vi "Prefilter_60Hz_Notch.vi"(8 "error in (no error)":errorcluster, 10 "Array in":waveform(dbl)[](array[waveform])) -> (0 "error out":errorcluster, 2 "Array out":waveform(dbl)[](array[waveform]))   [LabVIEW 2016, in "LockinDAQ.lvclass"]
uses:
  LockinDAQ.lvclass
  <vilib>/addons/Digital Filter Design/Design.llb/DFD IIR Notch Peak Design by Q.vi
  <vilib>/addons/Digital Filter Design/Process.llb/DFD Filtering (Wfm NChan).vi
  <vilib>/addons/Digital Filter Design/NI_DigFilterLicensed.lvlib
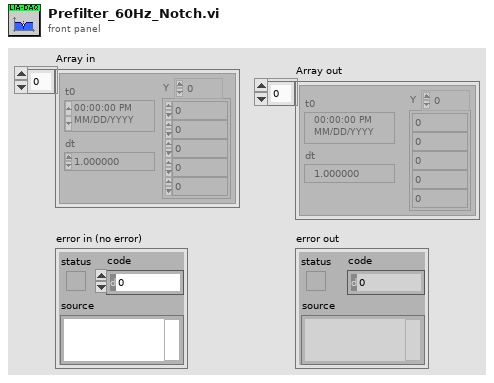
[diagram p1: front panel]
types:
  T1 = typedef "NI_DigFilterLicensed.lvlib/DFD Filter Obj.ctl" = cluster{"mSRate_Fs":dbl, "mSRate_Version":string, "mSRate_Comments":string, "mSRate_OrgCoef":T2, "mSRate_CurCoef":T2, "mSRate_Quantized?":bool, "mSRate_QCoef":T2, "mSRate_QSettings":T4[], "mSRate_Order":i32, "mSRate_Scaling":cluster{"mSRate_ScaleByPowerOf2?":bool, "mSRate_ScaleType":T6}}
  T2 = typedef "NI_DigFilterLicensed.lvlib/DFD Filter Coef.ctl" = cluster{"type":T3, "gain":dbl, "coef a (k)":dbl[], "coef b (v)":dbl[]}
  T3 = typedef "NI_DigFilterLicensed.lvlib/DFD Filter Structure Type Selector.ctl" = enum16{"Undefined", "FIR Direct Form", "FIR Direct Form Transposed", "FIR Symmetric", "FIR Antisymmetric", "IIR Direct Form I", "IIR Direct Form I Transposed", "IIR Direct Form II", "IIR Direct Form II Transposed", "IIR Cascaded Second Order Sections Form I", "IIR Cascaded Second Order Sections Form I Transposed", "IIR Cascaded Second Order Sections Form II", "IIR Cascaded Second Order Sections Form II Transposed", "Lattice Allpass (basic sections)", "Lattice Allpass (one multiplier sections)", "Lattice Allpass (normalized sections)", "Lattice AR (basic sections)", "Lattice AR (one multiplier sections)", "Lattice AR (normalized sections)", "Lattice MA (minimum phase)", "Lattice MA (maximum phase)", "Lattice ARMA (basic sections)", "Lattice ARMA (one multiplier sections)", "Lattice ARMA (normalized sections)"}
  T4 = typedef "NI_DigFilterLicensed.lvlib/dfd_Internal Quantization Settings.ctl" = cluster{"source":T5, "wl":i16, "iwl":i16, "overflow mode":enum16{"Saturation", "Wrap"}, "rounding mode":enum16{"Nearest", "Truncation"}, "signed?":bool}
  T5 = typedef "NI_DigFilterLicensed.lvlib/dfd_Internal Quantization Srcs.ctl" = u16
  T6 = typedef "NI_DigFilterLicensed.lvlib/DFD Coef Norm Type.ctl" = enum16{"No Norm", "Time Domain 1-Norm", "Time Domain 2-Norm", "Time Domain Inf-Norm"}
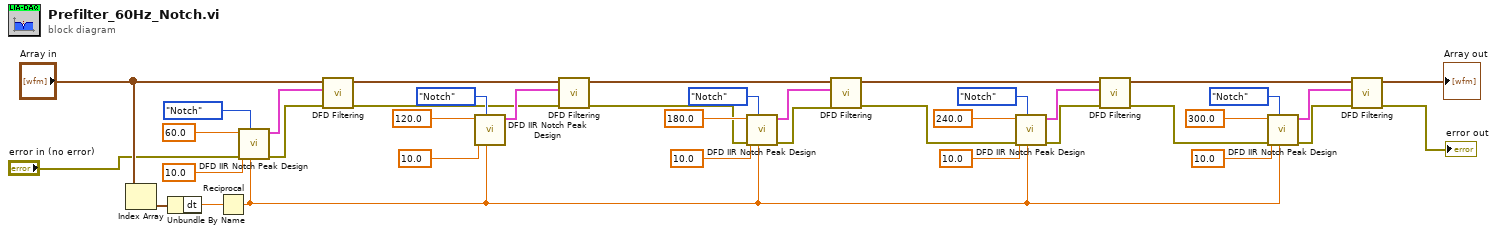
[diagram p0: block diagram]
diagram:
  n1 = Index Array(array="Array in") -> (element=w35:waveform(dbl))  [unwired: 1 in]
  n2 = Unbundle By Name(w35) -> ("dt"=w38:dbl)
  n3 = Reciprocal(x=w38) -> (1/x=w11:dbl)
  n4 = call-poly <vilib>:"DFD IIR Notch Peak Design.vi"("fs [Hz]"=w11, "filter type"=enum16{"Notch", "Peak"}."Notch", "error in (no error)"="error in (no error)", "Q factor"=10.0, "f0 [Hz]"=60.0) -> ("error out"=w7:errorcluster, "filter out"=w37:T1)  [unwired: 5 in]
  n5 = call-poly <vilib>:"DFD Filtering.vi"("error in (no error)"=w7, "filter"=w37, "signal in"="Array in") -> ("error out"=w10:errorcluster, "signal out"=w30:waveform(dbl)[])  [unwired: 7 in]
  n6 = call-poly <vilib>:"DFD IIR Notch Peak Design.vi"("fs [Hz]"=w11, "filter type"=enum16{"Notch", "Peak"}."Notch", "Q factor"=10.0, "f0 [Hz]"=120.0) -> ("filter out"=w29:T1)  [unwired: 6 in, 1 out]
  n7 = call-poly <vilib>:"DFD Filtering.vi"("error in (no error)"=w10, "filter"=w29, "signal in"=w30) -> ("error out"=w9:errorcluster, "signal out"=w14:waveform(dbl)[])  [unwired: 7 in]
  n8 = call-poly <vilib>:"DFD IIR Notch Peak Design.vi"("fs [Hz]"=w11, "filter type"=enum16{"Notch", "Peak"}."Notch", "error in (no error)"=w9, "Q factor"=10.0, "f0 [Hz]"=180.0) -> ("error out"=w6:errorcluster, "filter out"=w27:T1)  [unwired: 5 in]
  n9 = call-poly <vilib>:"DFD Filtering.vi"("error in (no error)"=w6, "filter"=w27, "signal in"=w14) -> ("error out"=w5:errorcluster, "signal out"=w13:waveform(dbl)[])  [unwired: 7 in]
  n10 = call-poly <vilib>:"DFD IIR Notch Peak Design.vi"("fs [Hz]"=w11, "filter type"=enum16{"Notch", "Peak"}."Notch", "error in (no error)"=w5, "Q factor"=10.0, "f0 [Hz]"=240.0) -> ("error out"=w4:errorcluster, "filter out"=w20:T1)  [unwired: 5 in]
  n11 = call-poly <vilib>:"DFD Filtering.vi"("error in (no error)"=w4, "filter"=w20, "signal in"=w13) -> ("error out"=w3:errorcluster, "signal out"=w12:waveform(dbl)[])  [unwired: 7 in]
  n12 = call-poly <vilib>:"DFD IIR Notch Peak Design.vi"("fs [Hz]"=w11, "filter type"=enum16{"Notch", "Peak"}."Notch", "error in (no error)"=w3, "Q factor"=10.0, "f0 [Hz]"=300.0) -> ("error out"=w2:errorcluster, "filter out"=w19:T1)  [unwired: 5 in]
  n13 = call-poly <vilib>:"DFD Filtering.vi"("error in (no error)"=w2, "filter"=w19, "signal in"=w12) -> ("error out"=→"error out":errorcluster, "signal out"=→"Array out":waveform(dbl)[])  [unwired: 7 in]
